vi "ClassInstaller.vi"   [LabVIEW 2019]
panel:
  # "Hit Run To Install"
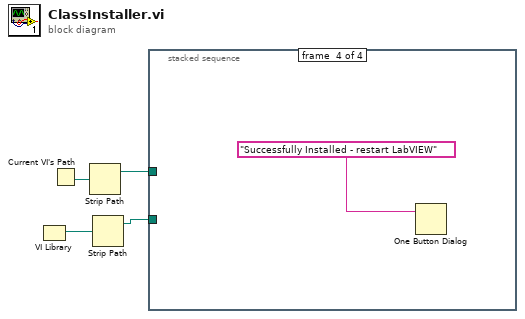
[diagram p0: block diagram]
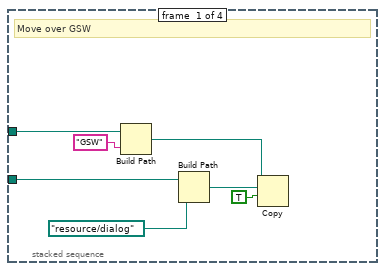
[diagram p2: hidden frame]
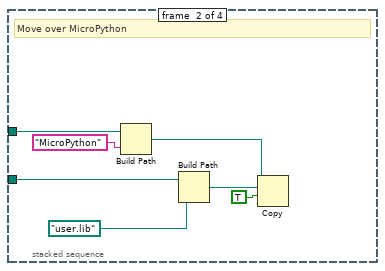
[diagram p3: hidden frame]
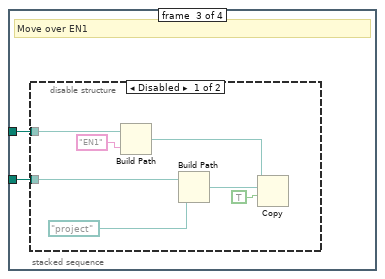
[diagram p4: hidden frame]
diagram:
  n1 = VI Library() -> (path=w2:path)
  n2 = Current VI's Path() -> (path=w4:path)
  n3 = Strip Path(path=w4) -> (stripped path=w3:path)  [unwired: 1 out]
  n4 = Strip Path(path=w2) -> (stripped path=w1:path)  [unwired: 1 out]
  n5 = stacked-sequence {
    tunnel: w3 -> [w9 w16 w20 _]
    tunnel: w1 -> [w5 w12 w19 _]
    frame #0 {
      # "Move over GSW"
      n6 = Build Path(base path=w9, name or relative path="GSW") -> (appended path=w6:path)
      n7 = Build Path(base path=w5, name or relative path=path "resource/dialog" ("Path")) -> (appended path=w7:path)
      n8 = Copy(9:TRUE ("overwrite (F)"), 10:w7, 11:w6) -> ()  [unwired: 2 in, 3 out]
    }
    frame #1 {
      # "Move over MicroPython"
      n9 = Build Path(base path=w16, name or relative path="MicroPython") -> (appended path=w13:path)
      n10 = Build Path(base path=w12, name or relative path=path "user.lib" ("Path")) -> (appended path=w14:path)
      n11 = Copy(9:TRUE ("overwrite (F)"), 10:w14, 11:w13) -> ()  [unwired: 2 in, 3 out]
    }
    frame #2 {
      # "Move over EN1"
      n12 = disable-structure shown="Disabled" {
        disable-tunnel: w20 -> [w25 _]
        disable-tunnel: w19 -> [w21 _]
        frame Disabled {
          n13 = Build Path(base path=w25, name or relative path="EN1") -> (appended path=w22:path)
          n14 = Build Path(base path=w21, name or relative path=path "project" ("Path")) -> (appended path=w23:path)
          n15 = Copy(9:TRUE ("overwrite (F)"), 10:w23, 11:w22) -> ()  [unwired: 2 in, 3 out]
        }
        frame Enabled {
        }
      }
    }
    frame #3 {
      n16 = One Button Dialog(message="Successfully Installed - restart LabVIEW") -> ()  [unwired: 1 in, 1 out]
    }
  }
